vi "PH_Stepmotor_BaseClass.Waveplate - Angle 2 Percent.vi"(1 "Angle [°]":dbl) -> (0 "rel. Intensity [%]":dbl format="%#.1f")   [LabVIEW 2014, in "PH_Stepmotor_BaseClass.lvlib"]
doc: "This VI calculalates the relative Intensity (in percent) for a given waveplate Angle (in degrees, coerced to the range between 0 and 45°) by\n\nrel. Intensity [%] = 100 * (sin (Angle [°] * 2))^2\n\nThe result is rounded to 1 digit after the decimal point."
uses:
  PH_Stepmotor_BaseClass.lvlib
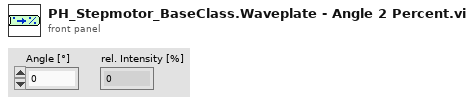
[diagram p1: front panel]
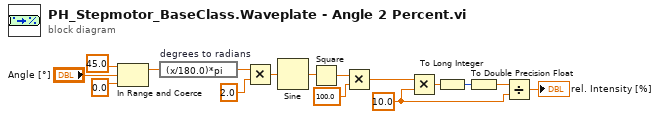
[diagram p0: block diagram]
diagram:
  w3 = 10.0 ("y")
  n1 = In Range and Coerce(upper limit=45.0, x="Angle [°]", lower limit=0.0) -> (coerced(x)=w9:dbl)  [unwired: 1 out]
  n2 = expression code="(x/180.0)*pi" "degrees to radians"(w9) -> (w15:dbl)
  n3 = Multiply(x=w15, y=2.0 ("Angle [°]")) -> (x*y=w13:dbl)
  n4 = Sine(x=w13) -> (sin(x)=w12:dbl)
  n5 = Square(x=w12) -> (x^2=w11:dbl)
  n6 = Multiply(x=w11, y=100.0) -> (x*y=w2:dbl)
  n7 = Multiply(x=w2, y=w3) -> (x*y=w6:dbl)
  n8 = To Long Integer(number=w6) -> (32bit integer=w5:i32)
  n9 = To Double Precision Float(number=w5) -> (double precision float=w4:dbl)
  n10 = Divide(x=w4, y=w3) -> (x/y=→"rel. Intensity [%]":dbl)
